vi "UI_CMPS12_I2C_Read.vi"() -> ()   [LabVIEW 2018]
uses:
  <vilib>/Rock Robotics/SystemInterfaces/i2clib/i2c_bus.ctl
panel:
  out "direction":dbl
  out "element":u8
  in  "stop":bool
  out "error out":errorcluster
  in  "error in":errorcluster
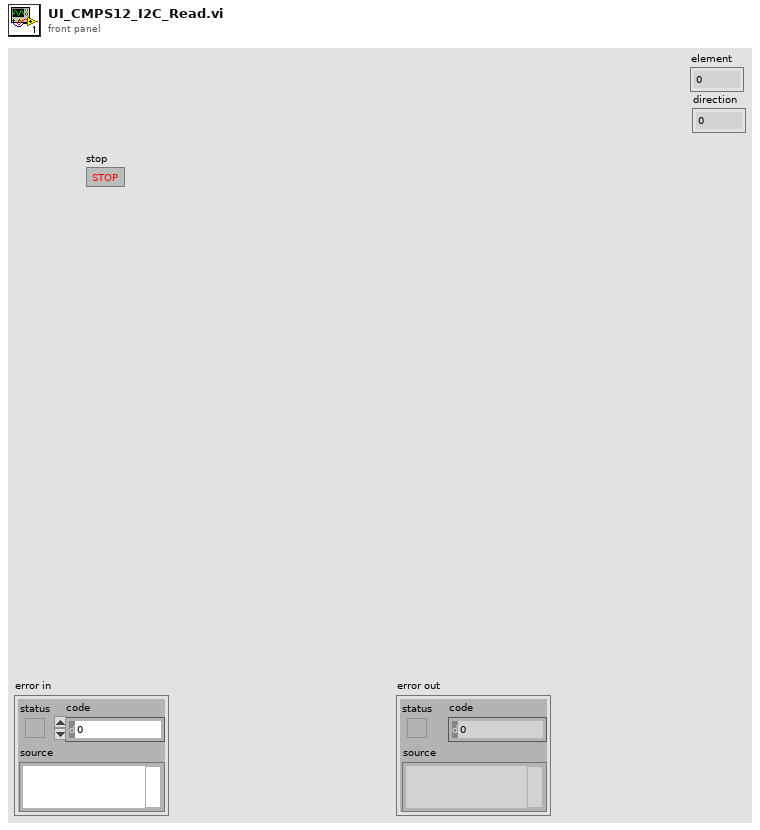
[diagram p1: front panel]
types:
  T1 = typedef "i2c_bus.ctl" = enum16{"I2C On-Board", "I2C MXP", "Invalid"}
  T2 = typedef "WPI_I2CDevRef.ctl" = cluster{"DevStatus":errorcluster, "Device Address":u8, "Handle":i32, "I2C Bus":T1}
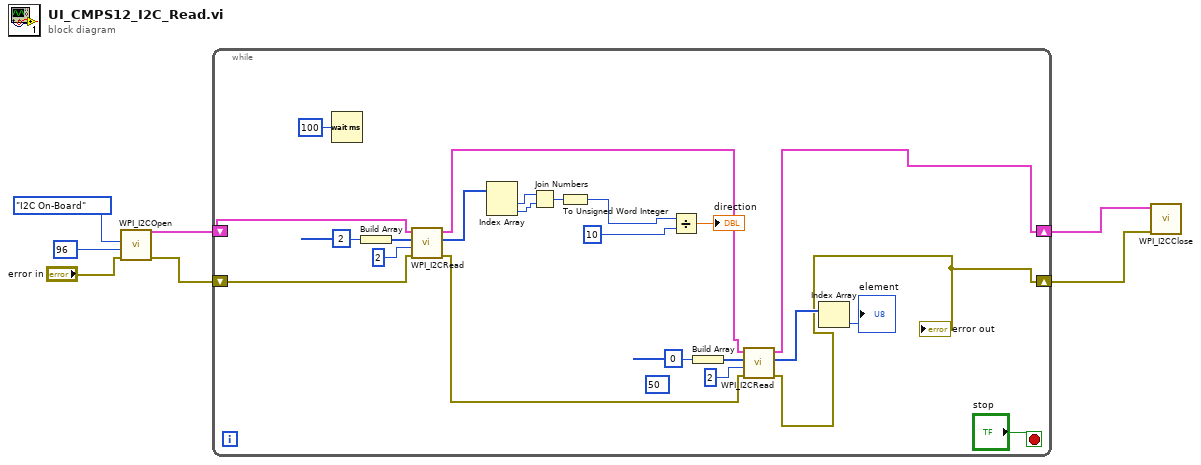
[diagram p0: block diagram]
diagram:
  n1 = call <vilib>:"WPI_I2COpen.vi"("error in"="error in", "Device Address"=u8 96 ("Data To Send"), "I2C Bus"=i2c_bus."I2C On-Board") -> ("error out"=w2:errorcluster, "I2CDevRef"=w4:T2)  [unwired: 1 in, 6 out]
  n2 = while {
    shift-right: [w11] -> w3
    shift-left: w4 -> [w26]
    shift-right: [w13] -> w1
    shift-left: w2 -> [w23]
    stop <- "stop" stop-if-true
    (unwired) u8 50 ("Data To Send")
    n3 = Wait (ms)(milliseconds to wait=u32 100) -> ()  [unwired: 1 out]
    n4 = Build Array(u8 2 ("Data To Send")) -> (w28:u8[])
    n5 = call <vilib>:"WPI_I2CRead.vi"("error in (no error)"=w23, "I2CBytesToRead"=u8 2, "I2CRegister"=w28, "I2CDevRef"=w26) -> ("error out"=w14:errorcluster, "Data Out"=w30:u8[], "I2CDevRef"=w12:T2)  [unwired: 5 out]
    n6 = Index Array(array=w30) -> (element #1=w21:u8, element #2=w20:u8)  [unwired: 2 in]
    n7 = Join Numbers(hi=w21, lo=w20) -> ((hi.lo)=w29:u16)
    n8 = To Unsigned Word Integer(number=w29) -> (unsigned 16bit integer=w10:u16)
    n9 = Divide(x=w10, y=u16 10) -> (x/y=→"direction":dbl)
    n10 = Build Array(u8 0 ("Data To Send")) -> (w17:u8[])
    n11 = call <vilib>:"WPI_I2CRead.vi"("error in (no error)"=w14, "I2CBytesToRead"=u8 2, "I2CRegister"=w17, "I2CDevRef"=w12) -> ("error out"=w13:errorcluster, "Data Out"=w16:u8[], "I2CDevRef"=w11:T2)  [unwired: 5 out]
    "error out" <- w13
    n12 = Index Array(array=w16) -> (element=→"element":u8)  [unwired: 1 in]
  }
  n13 = call <vilib>:"WPI_I2CClose.vi"("error in (no error)"=w1, "I2CDevRef"=w3) -> ()  [unwired: 9 in, 1 out]
